vi "whisky.vi"(5 "Median":dbl format="%.2f", 6 "Lower Quartile (LQ)":dbl format="%.4f", 7 "Upper Quartile (UQ)":dbl format="%.4f") -> (0 "L2":dbl format="%.4f", 1 "L1":dbl format="%.4f", 2 "U1":dbl format="%.4f", 3 "U2":dbl format="%.4f")   [LabVIEW 2021, in "statistics.lvlib"]
uses:
  statistics.lvlib
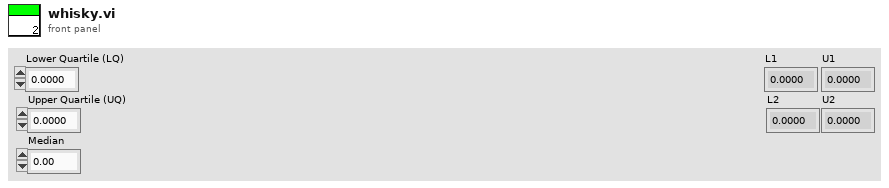
[diagram p1: front panel]
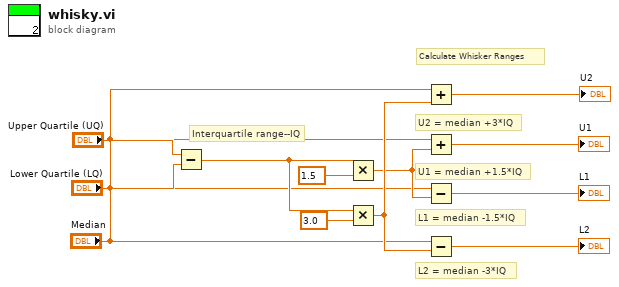
[diagram p0: block diagram]
diagram:
  # "L1 = median -1.5*IQ"
  # "Interquartile range--IQ"
  # "L2 = median -3*IQ"
  # "U1 = median +1.5*IQ"
  # "U2 = median +3*IQ"
  # "Calculate Whisker Ranges"
  n1 = Subtract(x="Upper Quartile (UQ)", y="Lower Quartile (LQ)") -> (x-y=w6:dbl)
  n2 = Multiply(x=w6, y=1.5) -> (x*y=w5:dbl)
  n3 = Multiply(x=w6, y=3.0) -> (x*y=w8:dbl)
  n4 = Add(x="Median", y=w8) -> (x+y=→"U2":dbl)
  n5 = Add(x="Median", y=w5) -> (x+y=→"U1":dbl)
  n6 = Subtract(x="Median", y=w5) -> (x-y=→"L1":dbl)
  n7 = Subtract(x="Median", y=w8) -> (x-y=→"L2":dbl)
